vi "CloseHandler.vi"(8 "error in (no error)":errorcluster, 11 "DataHandling in":refnum<class "DataHandlerMYiTOPS.lvclass">) -> (0 "error out":errorcluster, 3 "DataHandling out":refnum<class "DataHandlerMYiTOPS.lvclass">)   [LabVIEW 2017, in "DataHandlerMYiTOPS.lvclass"]
uses:
  DataHandlerMYiTOPS.lvclass
  DataHandlerMYiTOPS.lvclass/DataHandlerMYiTOPS.ctl
  <vilib>/drjdpowell/SQLite Library/SQL Connection/Connection.lvclass
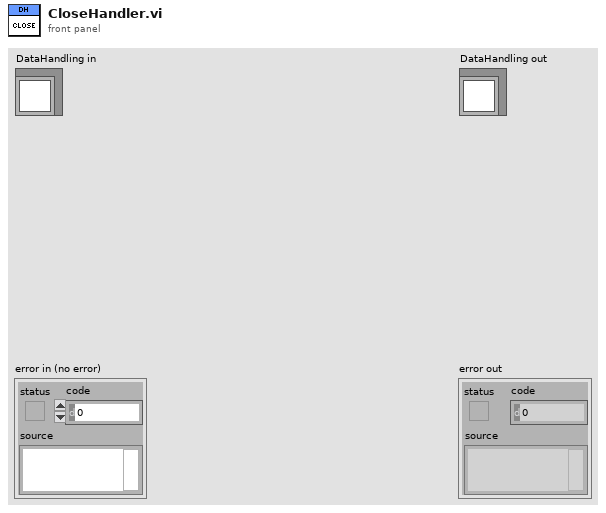
[diagram p1: front panel]
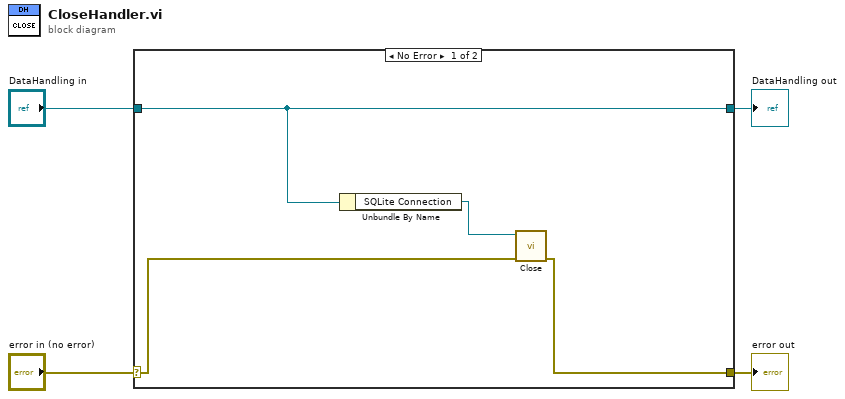
[diagram p0: block diagram]
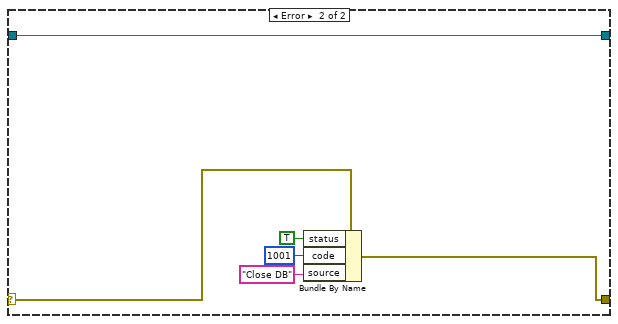
[diagram p2: hidden frame]
diagram:
  n1 = case shown="No Error" "error in (no error)" {
    selector: "error in (no error)" -> [w6 w13]
    tunnel: [w5 w12] -> w3
    tunnel: [w7 w14] -> w1
    tunnel: "DataHandling in" -> [w7 w14]
    frame No Error {
      n2 = Unbundle By Name(w7) -> ("SQLite Connection"=w8:refnum<class "Connection.lvclass">)
      n3 = call-dynamic "Close.vi"("error in (no error)"=w6, "SQLite Connection in"=w8) -> ("error out"=w5:errorcluster)  [unwired: 9 in]
    }
    frame Error {
      n4 = Bundle By Name(cluster=w13, "status"=TRUE, "code"=1001, "source"="Close DB") -> (w12:errorcluster)
    }
  }
  "error out" <- w3
  "DataHandling out" <- w1
